vi "Load Component User Interfaces.vi"(8 "error in (no error)":errorcluster, 10 "component names":string[](array[string]), 11 "Component Loader in":refnum<class "Component Loader.lvclass">) -> (0 "error out":errorcluster, 2 "Component UIs":refnum<class "Component User Interfaces.lvclass">[](array[class]), 3 "Component Loader out":refnum<class "Component Loader.lvclass">)   [LabVIEW 2019, in "DSF Core.lvlib" / "Component Loader.lvclass"]
uses:
  Component Loader.lvclass
  Component User Interface/Component User Interfaces.lvclass
  Component/Component.lvclass
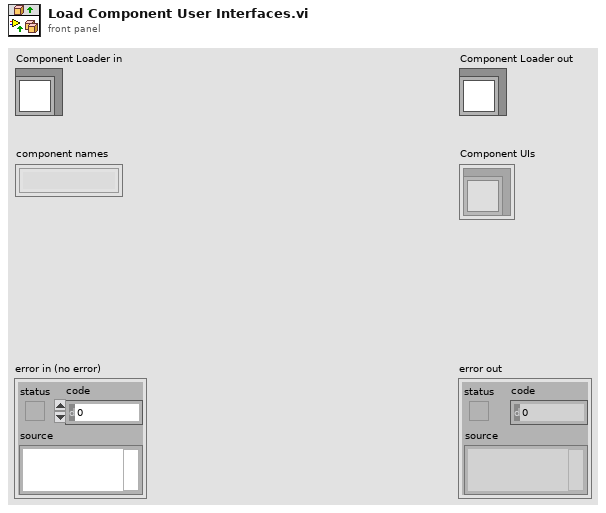
[diagram p1: front panel]
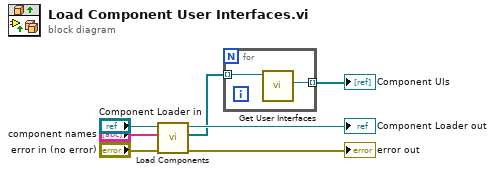
[diagram p0: block diagram]
diagram:
  n1 = call "Load Components.vi"("error in (no error)"="error in (no error)", "component names"="component names", "Component Loader in"="Component Loader in") -> ("error out"=→"error out":errorcluster, "Components"=w1:refnum<class "Component.lvclass">[], "Component Loader out"=→"Component Loader out":refnum<class "Component Loader.lvclass">)  [unwired: 6 in]
  n2 = for {
    tunnel: w1 -> [w9] mode=indexing
    tunnel: [w8] -> w2 mode=indexing
    n3 = call "Get User Interfaces.vi"("Component in"=w9) -> ("User Interfaces"=w8:refnum<class "Component User Interfaces.lvclass">)  [unwired: 9 in, 1 out]
  }
  "Component UIs" <- w2
